vi "Test cases.vi"(2 "Total number of cases\nin the input file is:":i32=10) -> (4 "Continue? (T=yes)":bool=TRUE, 6 "Test cases":i32)   [LabVIEW 2010]
panel:
  out "Total number of cases\nin the input file is:":i32=10
  out "Training cases (%)":i32=100
  out "Test cases (%)":i32
  in  "Test cases:":i32
  out "Training cases:":i32=10
  in  "Exit":bool
  in  "OK":bool
  # "How many test cases?"
  # "100%"
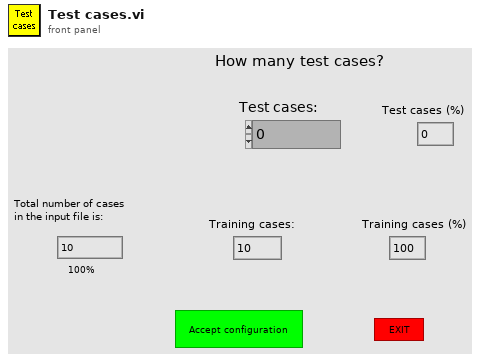
[diagram p1: front panel]
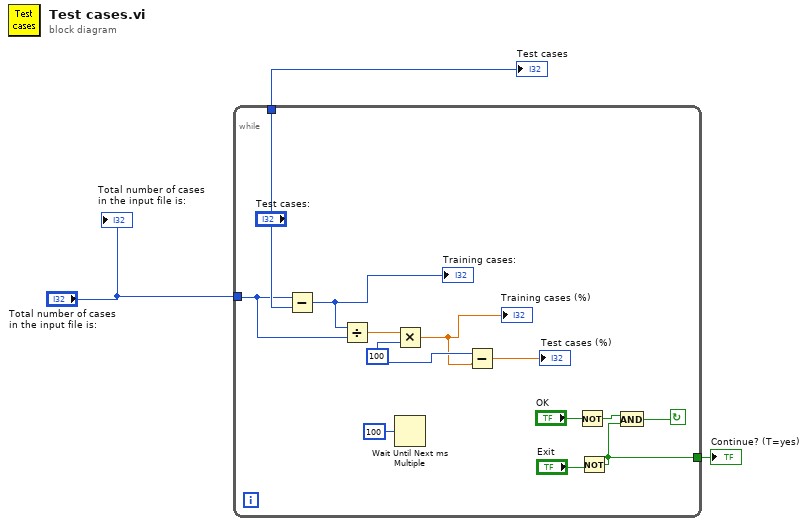
[diagram p0: block diagram]
diagram:
  n1 = while {
    tunnel: ["Test cases:"] -> w1
    tunnel: "Total number of cases\nin the input file is:" -> [w9]
    tunnel: [w12] -> w3
    stop <- w13 continue-if-true
    w7 = 100
    n2 = Subtract(x=w9, y="Test cases:") -> (x-y=w6:i32)
    "Training cases:" <- w6
    n3 = Divide(x=w6, y=w9) -> (x/y=w8:dbl)
    n4 = Multiply(x=w8, y=w7) -> (x*y=w5:dbl)
    "Training cases (%)" <- w5
    n5 = Wait Until Next ms Multiple(millisecond multiple=u32 100) -> ()  [unwired: 1 out]
    n6 = Subtract(x=w7, y=w5) -> (x-y=→"Test cases (%)":dbl)
    n7 = Not(x="OK") -> (.not. x?=w15:bool)
    n8 = Not(x="Exit") -> (.not. x?=w12:bool)
    n9 = And(x=w15, y=w12) -> (x .and. y?=w13:bool)
  }
  "Continue? (T=yes)" <- w3
  "Test cases" <- w1
  "Total number of cases\nin the input file is:" <- "Total number of cases\nin the input file is:"
